vi "LinearSystemSim_New.vi"(9 "MeasurementStdDev":T1, 11 "System":T2) -> (0 "Size Coerced":bool, 3 "LinearSystemSim":T3)   [LabVIEW 2019, in "Trajectory_Library.lvlib"]
doc: "Creates a simulated generic linear system with measurement noise.\n\nThis class helps simulate linear systems. \n\nCall setInput(double...)} with the inputs to the system (usually voltage).\n\nCall update to update the simulation.\n\nSet simulated sensor readings with the simulated positions in getOutput(). (Outputs of the simulation are inputs to the robot -- sensors.)\n \nInputs:\n - system -- The Linear System being controlled.\n - measurementStdDevs -- Standard deviations of measurements. Can be null if no noise is desired.\n\nOutputs:\n - OutLinearSystemSim -- Updated data cluster\n - Error -- If TRUE, an error occured."
uses:
  Trajectory_Library.lvlib
  <vilib>/Analysis/Matrix/Datatypes/RealMatrix.ctl
  <vilib>/Analysis/Matrix/NI_Matrix.lvlib
  TypeDef/LINEAR_SYSTEM.ctl
  TypeDef/LINEAR_SYSTEM_SIM.ctl
panel:
  # "<States,States>"
  # "<States,Inputs>"
  # "<Outputs,States>"
  # "<Outputs,Inputs>"
  # "<States, 1>"
  # "<Outputs, 1>"
  # "<Inputs, 1>"
  # "<Outputs, 1>"
  # "<States,States>"
  # "<States,Inputs>"
  # "<Outputs,States>"
  # "<Outputs,Inputs>"
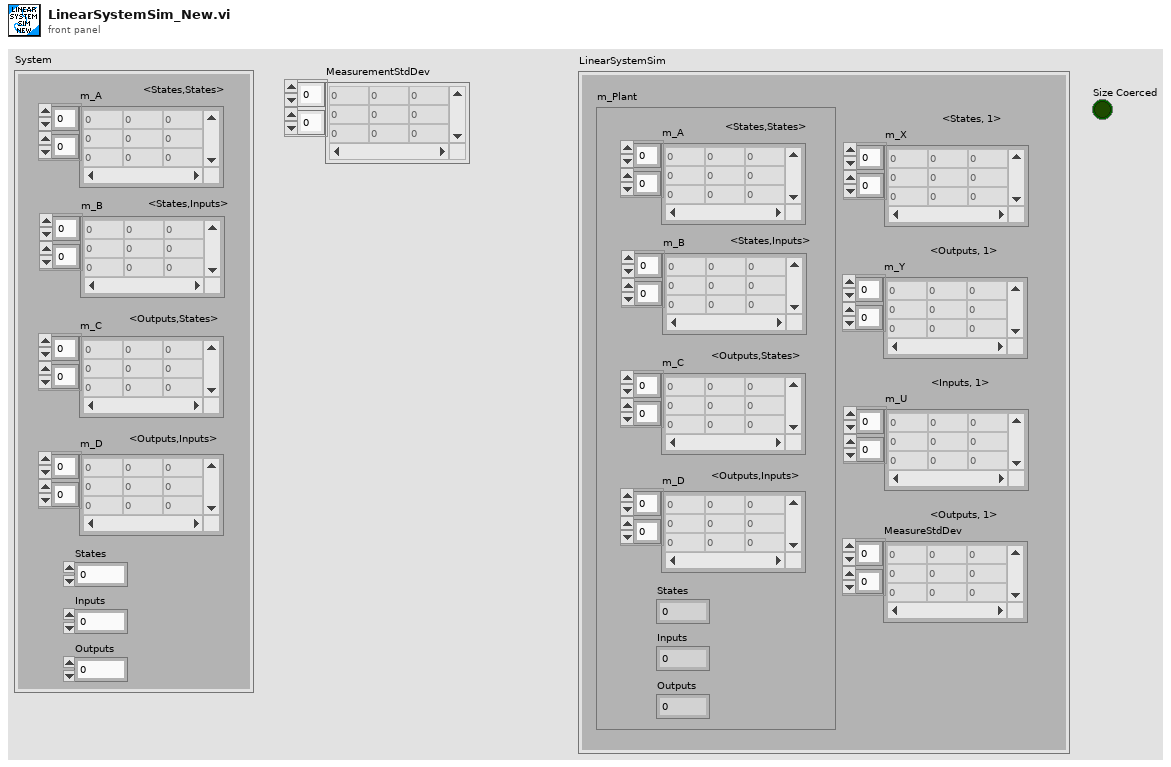
[diagram p1: front panel]
types:
  T1 = typedef "NI_Matrix.lvlib/RealMatrix.ctl" = dbl[][]
  T2 = typedef "Trajectory_Library.lvlib/LINEAR_SYSTEM.ctl" = cluster{"m_A":T1, "m_B":T1, "m_C":T1, "m_D":T1, "States":i32, "Inputs":i32, "Outputs":i32}
  T3 = typedef "Trajectory_Library.lvlib/LINEAR_SYSTEM_SIM.ctl" = cluster{"m_Plant":T2, "m_X":T1, "m_Y":T1, "m_U":T1, "MeasureStdDev":T1}
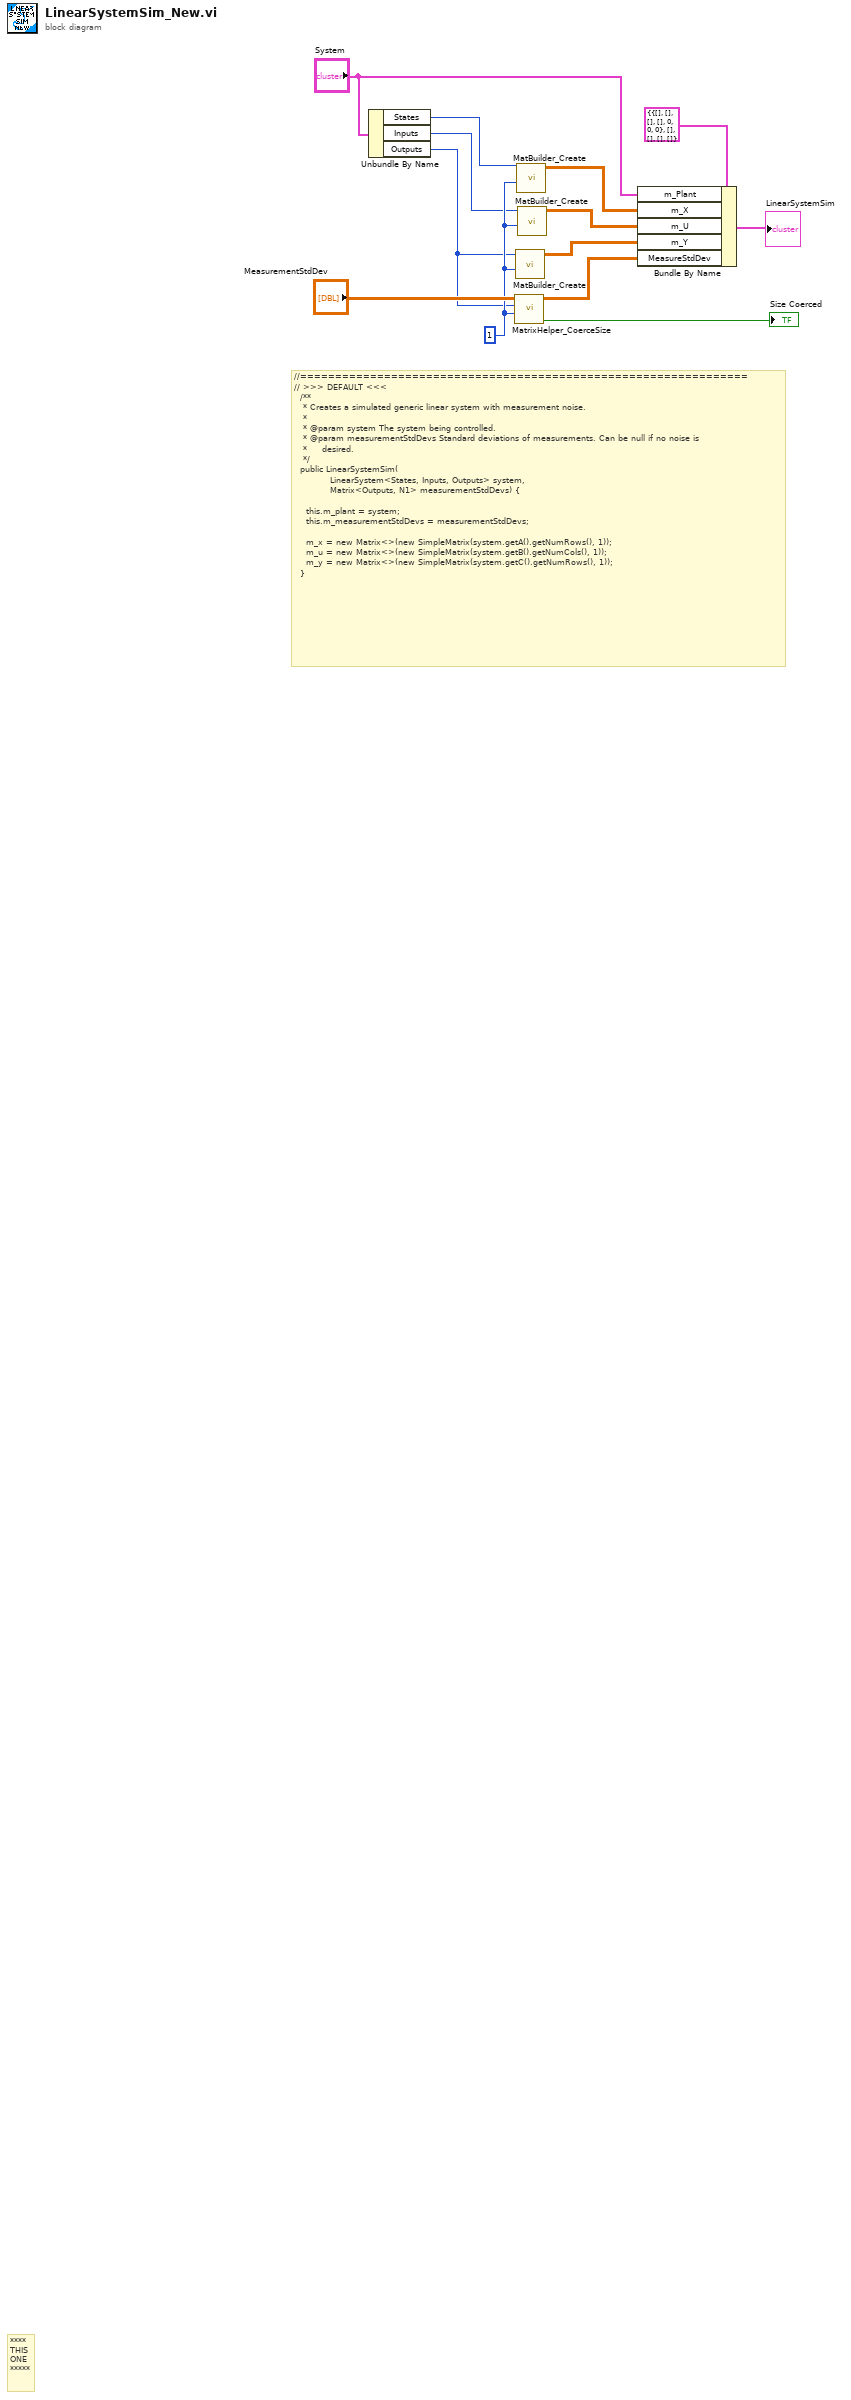
[diagram p0: block diagram]
diagram:
  w7 = 1 ("Columns")
  # "//================================================================\n// >>> DEFAULT <<<\n  /**\n   * Creates a simulated generic linear system with measurement noise.\n   *\n   * @param system The system being controlled.\n   * @param measurementStdDevs Standard deviations of measurements. Can be null if no noise is\n   *     desired.\n   */\n  public LinearSystemSim(\n           \tLinearSystem<States, Inputs, Outputs> system, \n\t           Matrix<Outputs, N1> measurementStdDevs) {\n\n    this.m_plant = system;\n    this.m_measurementStdDevs = measurementStdDevs;\n\n    m_x = new Matrix<>(new SimpleMatrix(system.getA().getNumRows(), 1));\n    m_u = new Matrix<>(new SimpleMatrix(system.getB().getNumCols(), 1));\n    m_y = new Matrix<>(new SimpleMatrix(system.getC().getNumRows(), 1));\n  }"
  # "****\nTHIS\nONE\n*****"
  n1 = Unbundle By Name("System") -> ("States"=w8:i32, "Inputs"=w5:i32, "Outputs"=w3:i32)
  n2 = call "MatrixHelper_CoerceSize.vi"("Columns"=w7, "Rows"=w3, "input matrix"="MeasurementStdDev") -> ("Coerced"=→"Size Coerced":bool, "output matrix"=w10:T1)  [unwired: 7 in]
  n3 = call "MatBuilder_Create.vi"("Columns"=w7, "Rows"=w3) -> ("output matrix"=w2:T1)  [unwired: 9 in]
  n4 = call "MatBuilder_Create.vi"("Columns"=w7, "Rows"=w8) -> ("output matrix"=w6:T1)  [unwired: 9 in]
  n5 = call "MatBuilder_Create.vi"("Columns"=w7, "Rows"=w5) -> ("output matrix"=w4:T1)  [unwired: 9 in]
  n6 = Bundle By Name(cluster=T3 {"m_Plant"={"m_A"=[], "m_B"=[], "m_C"=[], "m_D"=[], "States"=0, "Inputs"=0, "Outputs"=0}, "m_X"=[], "m_Y"=[], "m_U"=[], "MeasureStdDev"=[]} ("LINEAR_SYSTEM_SIM"), "m_Plant"="System", "m_X"=w6, "m_U"=w4, "m_Y"=w2, "MeasureStdDev"=w10) -> (→"LinearSystemSim":T3)
